vi "HAPS_PhaseSweep_Preamp(Hz)_allON.vi"() -> ()   [LabVIEW 2023, in "HAPS.lvlib"]
uses:
  HAPS.lvlib
  MCU_Function.ctl
  set_ele.ctl
  HAPS_SerialPort.ctl
  HAPS_MCU_ELE_Func.ctl
  R_S/R_S.lvlib
panel:
  in  "IC_On/OFF":bool[][](array[boolean])=[[TRUE, TRUE, TRUE, TRUE, TRUE, TRUE, FALSE, FALSE, FALSE, FALSE, FALSE, FALSE, TRUE], [FALSE, FALSE, FALSE, FALSE, FALSE, FALSE, FALSE, FALSE, FALSE, FALSE, FALSE, FALSE, FALSE], [FALSE, FALSE, FALSE, FALSE, FALSE, FALSE, TRUE, TRUE, TRUE, TRUE, TRUE, FALSE, TRUE]]
  in  "comn_gain":i32=17
  in  "ele_gain":i32=35
  in  "File_note":string
  in  "Init?":bool=TRUE
  out "Duration":dbl
  out "In-Phase : Phase(degree)":dbl[](graph)
  out "In-Phase : Gain(dB)":dbl[](graph)
  out "channel":i32
  out "chain_id":i32
  out "group":i32
  out "array_id":i32
  in  "Tx/Rx":enum16{"Rx", "Tx"}(ring)=enum."Tx"
  in  "array_id (MCU index)":i32
  in  "MCU_UART_addr":refnum<visa-resource-name>="COM8"
  in  "Target(degree)":dbl format="%#_13g"
  in  "SweepPoints":i32=11
  in  "sParameter":i32=21
  in  "Stop_Freq(GHz)":i64=39000000250
  in  "Start_Freq(GHz)":i64=38999999750
  in  "VISA resource name":refnum<visa-resource-name>="TCPIP0::192.168.119.45::inst0::INSTR"
  in  "HAPS_Equipment":enum16{"Keysight", "R&S"}(ring)=enum."R&S"
  # "HAPS_24x24_Phase_Sweep_Preamp(Hz)_allON"
  # "VNA"
  # "DUT"
  # "Tx:35\nRx:22"
  # "4718.54"
  # "TCPIP0::192.168.1.31::hislip0::INSTR"
  # "Group_0"
  # "Group_1"
  # "Group_2"
  # "0"
  # "5"
  # "6"
  # "11"
  # "Test Status"
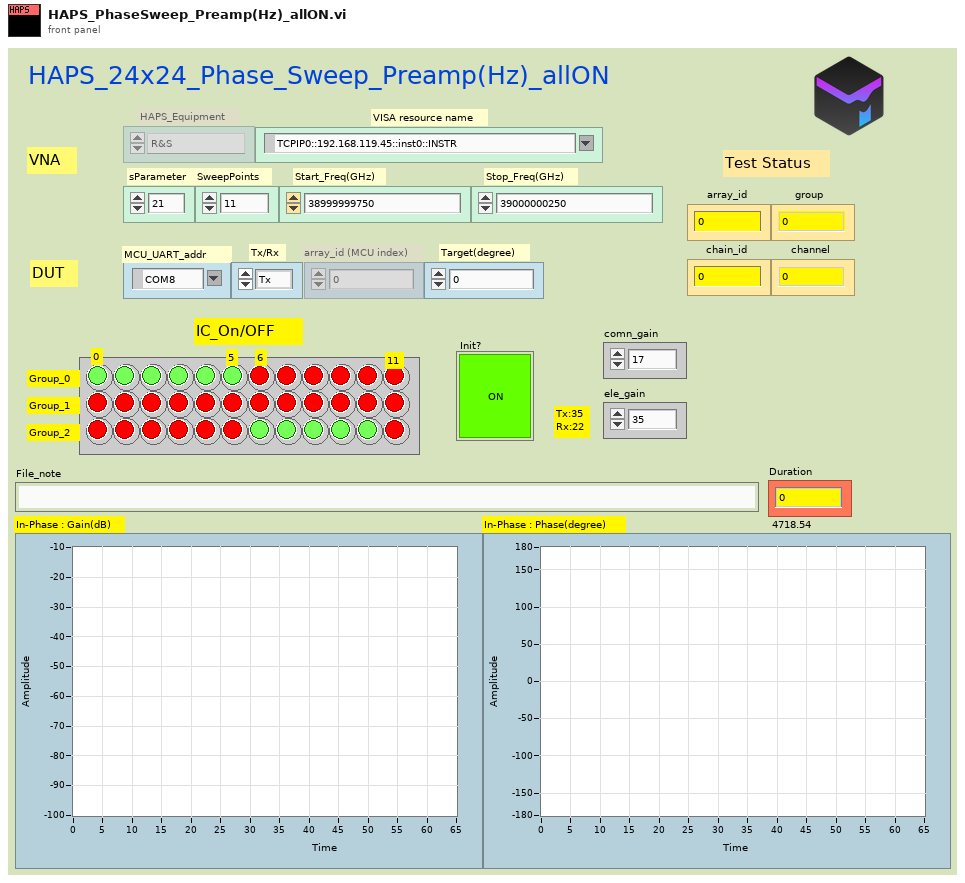
[diagram p1: front panel]
types:
  T1 = typedef "HAPS.lvlib/HAPS_SerialPort.ctl" = enum16{"Init", "Close", "CMD", "Flush"}
  T2 = typedef "HAPS.lvlib/HAPS_MCU_ELE_Func.ctl" = enum16{"array_init", "set_com_gain", "set_ch_gain_phase", "set_pd_range", "get_preamp_temp", "get_bfic_temp", "get_tx_pd", "ch_on", "ch_on_2", "ch_ctrl_all", "array_ctrl_src"}
  T3 = typedef "HAPS.lvlib/MCU_Function.ctl" = cluster{"Tx/Rx":enum16{"Rx", "Tx"}, "Enable?":enum16{"OFF", "On"}, "Source":enum16{"MCU", "ACU"}}
  T4 = typedef "HAPS.lvlib/set_ele.ctl" = cluster{"ch":i32, "chain_id":i32, "group":i32, "array_id":i32, "ele_phase":i32, "ele_gain":i32, "com_gain":i32, "pd_range":i32}
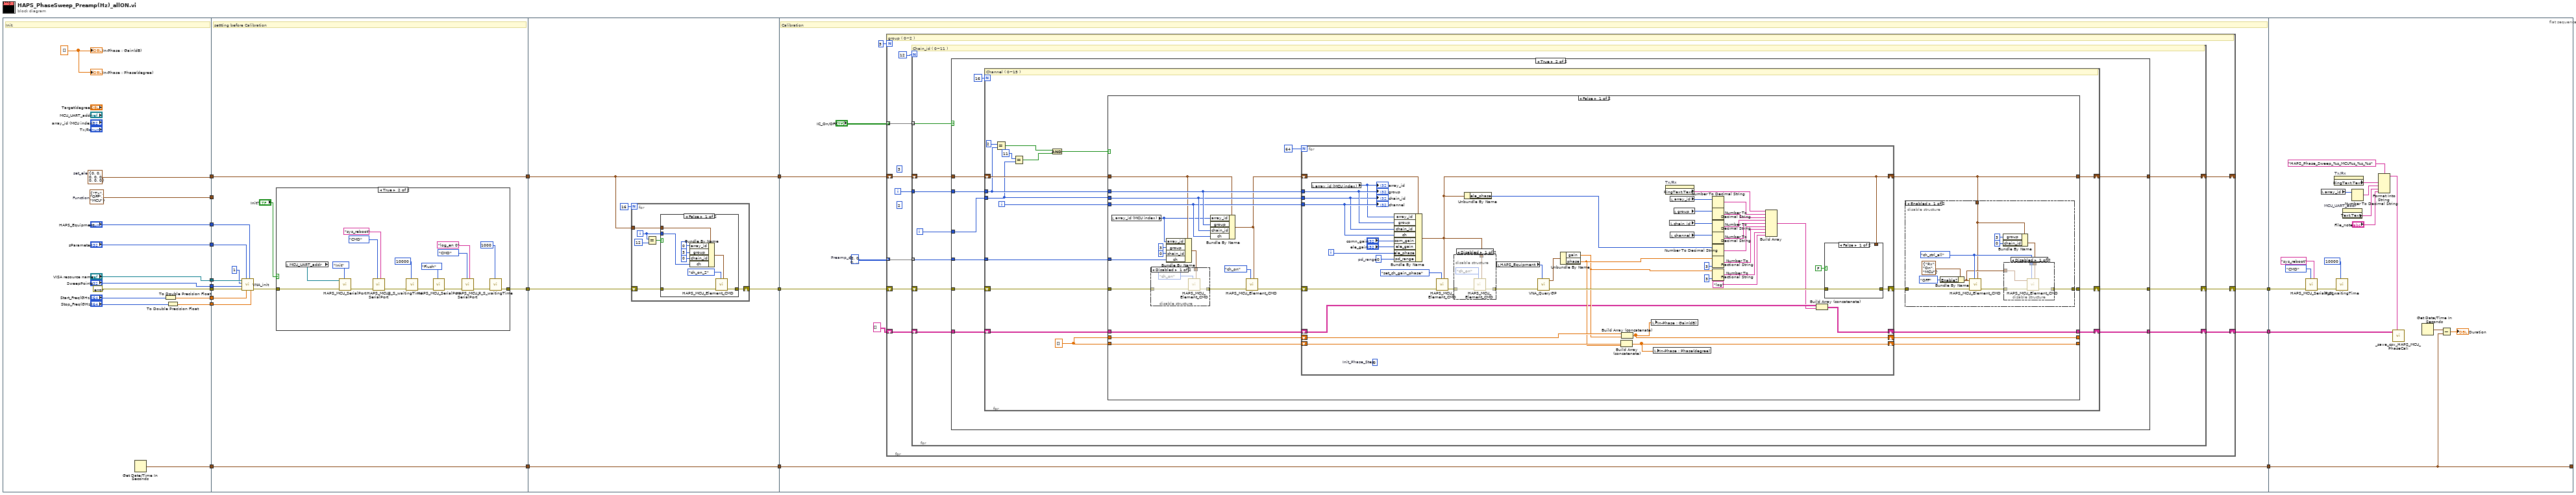
[diagram p0: block diagram]
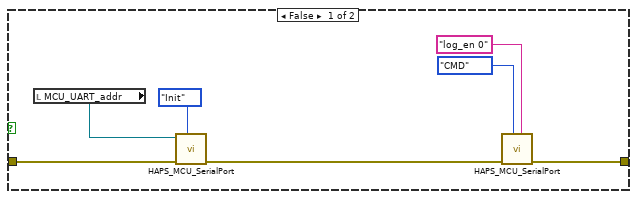
[diagram p2: hidden frame]
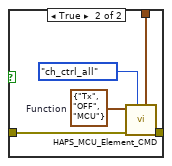
[diagram p9: hidden frame]
diagram:
  n1 = flat-sequence {
    tunnel: [w25] -> w19
    tunnel: [w32] -> w18
    tunnel: [errorcluster {"status"=FALSE, "code"=0, "source"=""} ("error in")] -> w17
    tunnel: ["sParameter"] -> w16
    tunnel: ["VISA resource name"] -> w15
    tunnel: [w21] -> w14
    tunnel: [w20] -> w13
    tunnel: ["SweepPoints"] -> w12
    tunnel: ["HAPS_Equipment"] -> w11
    tunnel: [w22] -> w10
    tunnel: w19 -> [w45]
    tunnel: w18 -> [_]
    tunnel: [w45] -> w6
    tunnel: w17 -> [w44]
    tunnel: [w36] -> w4
    tunnel: w16 -> [w43]
    tunnel: w15 -> [w42]
    tunnel: w14 -> [w41]
    tunnel: w13 -> [w40]
    tunnel: w12 -> [w39]
    tunnel: w11 -> [w35]
    tunnel: [w34] -> w2
    tunnel: w10 -> [w34]
    tunnel: w6 -> [w70]
    tunnel: [w70] -> w5
    tunnel: w4 -> [w71]
    tunnel: [w72] -> w3
    tunnel: w2 -> [w73]
    tunnel: [w73] -> w1
    tunnel: w5 -> [w97]
    tunnel: w3 -> [w98]
    tunnel: w1 -> [w94]
    tunnel: [w94] -> w9
    tunnel: [w93] -> w8
    tunnel: [w91] -> w7
    tunnel: [w262] -> _
    tunnel: w9 -> [w262]
    tunnel: w8 -> [w264]
    tunnel: w7 -> [w257]
    frame #0 {
      w23 = dbl[] []
      w25 = T4 {"ch"=0, "chain_id"=0, "group"=0, "array_id"=0, "ele_phase"=0, "ele_gain"=0, "com_gain"=0, "pd_range"=0}  # set_ele
      w32 = T3 {"Tx/Rx"=enum."Tx", "Enable?"=enum."OFF", "Source"=enum."MCU"}  # Function
      # "Init"
      n2 = Get Date/Time In Seconds() -> (seconds since 1Jan1904=w22:timestamp)
      n3 = To Double Precision Float(number="Start_Freq(GHz)") -> (double precision float=w21:dbl)
      n4 = To Double Precision Float(number="Stop_Freq(GHz)") -> (double precision float=w20:dbl)
      "In-Phase : Gain(dB)" <- w23
      "In-Phase : Phase(degree)" <- w23
    }
    frame #1 {
      # "settting before Calibration"
      n5 = call "VNA_init.vi"("Stop_Freq(GHz)"=w40, "HAPS_MCU_CMD"=w35, "Start_Freq(GHz)"=w41, "sParameter"=w43, "error in"=w44, "SweepPoints"=w39, "Mark no."=1, "VISA resource name"=w42) -> ("error out"=w37:errorcluster)  [unwired: 3 in]
      n6 = case shown="True" "Init?" {
        tunnel: w37 -> [w50 w66]
        tunnel: [w47 w53] -> w36
        frame False {
          n7 = local read "MCU_UART_addr"() -> (w48:refnum<visa-resource-name>)
          n8 = call "HAPS_MCU_SerialPort.vi"("HAPS_SerialPort_Func"=HAPS_SerialPort."Init", "error in"=w50, "VISA resource name"=w48) -> ("error out"=w46:errorcluster)  [unwired: 6 in, 2 out]
          n9 = call "HAPS_MCU_SerialPort.vi"("Command"="log_en 0", "HAPS_SerialPort_Func"=enum16{"Init", "Close", "CMD"}."CMD" ("HAPS_SerialPort"), "error in"=w46) -> ("error out"=w47:errorcluster)  [unwired: 6 in, 2 out]
        }
        frame True {
          n10 = local read "MCU_UART_addr"() -> (w64:refnum<visa-resource-name>)
          n11 = call "HAPS_MCU_SerialPort.vi"("HAPS_SerialPort_Func"=HAPS_SerialPort."Init", "error in"=w66, "VISA resource name"=w64) -> ("error out"=w61:errorcluster)  [unwired: 6 in, 2 out]
          n12 = call "HAPS_MCU_SerialPort.vi"("Command"="sys_reboot", "HAPS_SerialPort_Func"=enum16{"Init", "Close", "CMD"}."CMD" ("HAPS_SerialPort"), "error in"=w61) -> ("error out"=w60:errorcluster)  [unwired: 6 in, 2 out]
          n13 = call "R_S_waitingTime.vi"("Waiting Time(ms)"=u32 10000, "error in"=w60) -> ("error out"=w58:errorcluster)  [unwired: 9 in]
          n14 = call "HAPS_MCU_SerialPort.vi"("HAPS_SerialPort_Func"=HAPS_SerialPort."Flush", "error in"=w58) -> ("error out"=w56:errorcluster)  [unwired: 7 in, 2 out]
          n15 = call "HAPS_MCU_SerialPort.vi"("Command"="log_en 0", "HAPS_SerialPort_Func"=enum16{"Init", "Close", "CMD"}."CMD" ("HAPS_SerialPort"), "error in"=w56) -> ("error out"=w54:errorcluster)  [unwired: 6 in, 2 out]
          n16 = call "R_S_waitingTime.vi"("Waiting Time(ms)"=u32 1000, "error in"=w54) -> ("error out"=w53:errorcluster)  [unwired: 9 in]
        }
      }
    }
    frame #2 {
      n17 = for {
        N: 16 -> [_]
        shift-right: [w78] -> w72
        shift-left: w71 -> [w79]
        tunnel: w70 -> [w74]
        i -> [w76]
        n18 = Equal?(x=w76, y=12) -> (x = y?=w75:bool)
        n19 = case shown="False" w75 {
          tunnel: w79 -> [w83 w89]
          tunnel: [w82 w89] -> w78
          tunnel: w76 -> [w81 _]
          tunnel: w74 -> [w80 _]
          frame False {
            n20 = Bundle By Name(cluster=w80, "array_id"=0, "group"=3, "chain_id"=0, "ch"=w81) -> (w85:T4)
            n21 = call "HAPS_MCU_Element_CMD.vi"("set_ele"=w85, "HAPS_MCU_ELE_Func."=HAPS_MCU_ELE_Func."ch_on_2", "error in"=w83) -> ("error out"=w82:errorcluster)  [unwired: 7 in, 1 out]
          }
          frame True {
          }
        }
      }
    }
    frame #3 {
      w92 = i32[][] [[2, 0, 0, 8, 8, 10, 11, 9, 9, 1, 1, 3], [3, 1, 1, 9, 9, 11, 13, 15, 15, 7, 7, 5], [5, 7, 7, 15, 15, 13, 14, 14, 6, 6, 4, 12]]  # Preamp_ch
      # "Calibration"
      n22 = for {
        N: 3 -> [_]
        shift-right: [w108] -> _
        shift-left: w97 -> [w104]
        shift-right: [w107] -> w93
        shift-left: string[][] [] -> [w103]
        shift-right: [w106] -> w91
        shift-left: w98 -> [w105]
        tunnel: w92 -> [w100] mode=indexing
        tunnel: "IC_On/OFF" -> [w99] mode=indexing
        i -> [w101]
        (unwired) 2
        (unwired) 3
        # "group ( 0~2 )"
        n23 = for {
          N: 12 -> [_]
          shift-right: [w118] -> w108
          shift-left: w104 -> [w115]
          shift-right: [w117] -> w107
          shift-left: w103 -> [w114]
          shift-right: [w111] -> w106
          shift-left: w105 -> [w116]
          tunnel: w101 -> [w113]
          tunnel: w100 -> [w110] mode=indexing
          tunnel: w99 -> [w109] mode=indexing
          i -> [w112]
          # "Chain_id ( 0~11 )"
          n24 = case shown="True" w109 {
            tunnel: [w119 w130] -> w118
            tunnel: [w121 w129] -> w117
            tunnel: w116 -> [w120 w128]
            tunnel: w115 -> [w119 w127]
            tunnel: w114 -> [w121 w126]
            tunnel: w113 -> [_ w125]
            tunnel: w112 -> [_ w124]
            tunnel: [w120 w123] -> w111
            tunnel: w110 -> [_ w122]
            frame False {
            }
            frame True {
              n25 = for {
                N: 16 -> [_]
                shift-right: [w144] -> w130
                shift-left: w127 -> [w147]
                shift-right: [w142] -> w129
                shift-left: w126 -> [w143]
                shift-right: [w145] -> w123
                shift-left: w128 -> [w146]
                tunnel: w125 -> [w141]
                tunnel: w124 -> [w133]
                tunnel: w122 -> [w132]
                i -> [w134]
                w135 = dbl[] []
                # "Channel ( 0~15 )"
                n26 = Equal?(x=2, y=w141) -> (x = y?=w138:bool)
                n27 = Equal?(x=11, y=w133) -> (x = y?=w137:bool)
                n28 = And(x=w138, y=w137) -> (x .and. y?=w136:bool)
                n29 = case shown="False" w136 {
                  tunnel: w147 -> [w154 w251]
                  tunnel: w134 -> [w162 _]
                  tunnel: w146 -> [w155 w250]
                  tunnel: w141 -> [w164 _]
                  tunnel: w133 -> [w163 _]
                  tunnel: w135 -> [w171 w253]
                  tunnel: w135 -> [w170 w254]
                  tunnel: [w169 w253] -> _
                  tunnel: [w168 w254] -> _
                  tunnel: [w158 w250] -> w145
                  tunnel: [w157 w251] -> w144
                  tunnel: w143 -> [w166 w252]
                  tunnel: [w165 w252] -> w142
                  tunnel: w132 -> [w148 _]
                  frame False {
                    n30 = local read "array_id (MCU index)"() -> (w152:i32)
                    n31 = Bundle By Name(cluster=w154, "array_id"=w152, "group"=3, "chain_id"=0, "ch"=w148) -> (w153:T4)
                    n32 = disable-structure shown="Disabled" {
                      disable-tunnel: [w174 w176] -> w156
                      disable-tunnel: w155 -> [w173 w176]
                      disable-tunnel: w153 -> [w172 _]
                      frame Disabled {
                        n33 = call "HAPS_MCU_Element_CMD.vi"("set_ele"=w172, "HAPS_MCU_ELE_Func."=HAPS_MCU_ELE_Func."ch_on", "error in"=w173) -> ("error out"=w174:errorcluster)  [unwired: 7 in, 1 out]
                      }
                      frame Enabled {
                      }
                    }
                    n34 = Bundle By Name(cluster=w154, "array_id"=w152, "group"=w164, "chain_id"=w163, "ch"=w162) -> (w149:T4)
                    n35 = call "HAPS_MCU_Element_CMD.vi"("set_ele"=w149, "HAPS_MCU_ELE_Func."=HAPS_MCU_ELE_Func."ch_on", "error in"=w156) -> ("error out"=w160:errorcluster)  [unwired: 7 in, 1 out]
                    n36 = for {
                      N: 64 -> [_]
                      tunnel: w162 -> [w237]
                      tunnel: w164 -> [w235]
                      tunnel: w163 -> [w234]
                      shift-right: [w210] -> w169
                      shift-left: w171 -> [w212]
                      shift-right: [w209] -> w168
                      shift-left: w170 -> [w211]
                      shift-right: [w206] -> w159
                      shift-left: w160 -> [w236]
                      shift-right: [w196] -> w157
                      shift-left: w149 -> [w238]
                      shift-right: [w200] -> w165
                      shift-left: w166 -> [w202]
                      i -> [w208]
                      w232 = 0  # pd_range
                      (unwired) 0  # Init_Phase_Step
                      n37 = local read "array_id (MCU index)"() -> (w230:i32)
                      "array_id" <- w230
                      n38 = Bundle By Name(cluster=w238, "array_id"=w230, "group"=w235, "chain_id"=w234, "ch"=w237, "com_gain"="comn_gain", "ele_gain"="ele_gain", "ele_phase"=w208, "pd_range"=w232) -> (w196:T4)
                      n39 = call "HAPS_MCU_Element_CMD.vi"("set_ele"=w196, "HAPS_MCU_ELE_Func."=HAPS_MCU_ELE_Func."set_ch_gain_phase", "error in"=w236) -> ("error out"=w198:errorcluster)  [unwired: 7 in, 1 out]
                      n40 = disable-structure shown="Disabled" {
                        disable-tunnel: w198 -> [w242 w243]
                        disable-tunnel: [w241 w243] -> w197
                        disable-tunnel: w196 -> [w239 _]
                        frame Disabled {
                          n41 = call "HAPS_MCU_Element_CMD.vi"("set_ele"=w239, "HAPS_MCU_ELE_Func."=HAPS_MCU_ELE_Func."ch_on", "error in"=w242) -> ("error out"=w241:errorcluster)  [unwired: 7 in, 1 out]
                        }
                        frame Enabled {
                        }
                      }
                      n42 = Unbundle By Name(w196) -> ("ele_phase"=w205:i32)
                      n43 = local read "HAPS_Equipment"() -> (w214:enum16{"Keysight", "R&S"})
                      n44 = call "VNA_QueryGP.vi"("HAPS_Equipment"=w214, "error in"=w197) -> ("error out"=w207:errorcluster, "queryMarker"=w213:cluster{"gain":dbl, "phase":dbl})  [unwired: 8 in]
                      n45 = Unbundle By Name(w213) -> ("gain"=w203:dbl, "phase"=w204:dbl)
                      n46 = Build Array (concatenate)(w211, w204) -> (w209:dbl[])
                      n47 = Build Array (concatenate)(w212, w203) -> (w210:dbl[])
                      n48 = local write "In-Phase : Gain(dB)"(w210) -> ()
                      n49 = local write "In-Phase : Phase(degree)"(w209) -> ()
                      n50 = property on="Tx/Rx" class="Enum (strict)"() -> ("RingText.Text"=w219:string)  [unwired: 2 in, 2 out]
                      n51 = local read "chain_id"() -> (w216:i32)
                      n52 = local read "array_id"() -> (w218:i32)
                      n53 = local read "channel"() -> (w215:i32)
                      n54 = local read "group"() -> (w217:i32)
                      n55 = Number To Decimal String(number=w218) -> (decimal integer string=w220:string)  [unwired: 1 in]
                      n56 = Number To Decimal String(number=w217) -> (decimal integer string=w221:string)  [unwired: 1 in]
                      n57 = Number To Decimal String(number=w216) -> (decimal integer string=w222:string)  [unwired: 1 in]
                      n58 = Number To Decimal String(number=w215) -> (decimal integer string=w223:string)  [unwired: 1 in]
                      n59 = Number To Decimal String(number=w205) -> (decimal integer string=w224:string)  [unwired: 1 in]
                      n60 = Number To Fractional String(number=w204, precision (6)=i16 3) -> (F-format string=w227:string)  [unwired: 2 in]
                      n61 = Number To Fractional String(number=w203, precision (6)=i16 3) -> (F-format string=w228:string)  [unwired: 2 in]
                      n62 = Build Array(w219, w220, w221, w222, w223, w224, w227, w228, "log") -> (w201:string[])
                      n63 = Build Array (concatenate)(w202, w201) -> (w200:string[][])
                      n64 = case shown="False" FALSE {
                        tunnel: w207 -> [w244 w247]
                        tunnel: [w244 w246] -> w206
                        tunnel: w196 -> [_ w245]
                        frame False {
                        }
                        frame True {
                          w249 = T3 {"Tx/Rx"=enum."Tx", "Enable?"=enum."OFF", "Source"=enum."MCU"}  # Function
                          n65 = call "HAPS_MCU_Element_CMD.vi"("set_ele"=w245, "HAPS_MCU_ELE_Func."=HAPS_MCU_ELE_Func."ch_ctrl_all", "error in"=w247, "Function"=w249) -> ("error out"=w246:errorcluster)  [unwired: 6 in, 1 out]
                        }
                      }
                      "group" <- w235
                      "chain_id" <- w234
                      "channel" <- w237
                    }
                    n66 = disable-structure shown="Enabled" {
                      disable-tunnel: w159 -> [w187 w194]
                      disable-tunnel: [w183 w194] -> w158
                      disable-tunnel: w157 -> [w177 _]
                      frame Enabled {
                        w182 = HAPS_MCU_ELE_Func."ch_ctrl_all" ("HAPS_MCU_ELE_Func.")
                        n67 = Bundle By Name(cluster=T3 {"Tx/Rx"=enum."Rx", "Enable?"=enum."On", "Source"=enum."MCU"} ("Function"), "Enable?"=enum16{"OFF", "On"}."OFF") -> (w181:T3)
                        n68 = call "HAPS_MCU_Element_CMD.vi"("set_ele"=w177, "HAPS_MCU_ELE_Func."=w182, "error in"=w187, "Function"=w181) -> ("error out"=w184:errorcluster)  [unwired: 6 in, 1 out]
                        n69 = Bundle By Name(cluster=w177, "group"=3, "chain_id"=0) -> (w178:T4)
                        n70 = disable-structure shown="Disabled" {
                          disable-tunnel: w184 -> [w192 w193]
                          disable-tunnel: [w191 w193] -> w183
                          disable-tunnel: w182 -> [w190 _]
                          disable-tunnel: w181 -> [w189 _]
                          disable-tunnel: w178 -> [w188 _]
                          frame Disabled {
                            n71 = call "HAPS_MCU_Element_CMD.vi"("set_ele"=w188, "HAPS_MCU_ELE_Func."=w190, "error in"=w192, "Function"=w189) -> ("error out"=w191:errorcluster)  [unwired: 6 in, 1 out]
                          }
                          frame Enabled {
                          }
                        }
                      }
                      frame Disabled {
                      }
                    }
                  }
                  frame True {
                  }
                }
              }
            }
          }
        }
      }
    }
    frame #4 {
      n72 = call "HAPS_MCU_SerialPort.vi"("Command"="sys_reboot", "HAPS_SerialPort_Func"=enum16{"Init", "Close", "CMD"}."CMD" ("HAPS_SerialPort"), "error in"=w257) -> ("error out"=w255:errorcluster)  [unwired: 6 in, 2 out]
      n73 = local read "array_id"() -> (w267:i32)
      n74 = property on="Tx/Rx" class="Enum (strict)"() -> ("RingText.Text"=w266:string)  [unwired: 2 in, 2 out]
      n75 = call "R_S_waitingTime.vi"("Waiting Time(ms)"=u32 10000, "error in"=w255) -> ()  [unwired: 9 in, 1 out]
      n76 = property on="MCU_UART_addr" class="VISAName"() -> ("Text.Text"=w270:string)  [unwired: 2 in, 2 out]
      n77 = Number To Decimal String(number=w267) -> (decimal integer string=w268:string)  [unwired: 1 in]
      n78 = Format Into String(format string="HAPS_Phase_Sweep_%s_MCU%s_%s_%s", w266, w268, w270, "File_note") -> (resulting string=w269:string)  [unwired: 2 in, 1 out]
      n79 = call "_save_csv_HAPS_MCU_PhaseCali.vi"("NoteName"=w269, "array in"=w264) -> ()  [unwired: 9 in, 1 out]
      n80 = Get Date/Time In Seconds() -> (seconds since 1Jan1904=w263:timestamp)
      n81 = Subtract(x=w263, y=w262) -> (x-y=→"Duration":dbl)
    }
  }
